vi "DAQ.44xx.Get Ref Clk.vi"(8 "error in (no error)":errorcluster, 11 "Refnum in":refnum<k21>) -> (0 "error out":errorcluster, 2 "RefClk.Src":tag, 3 "Refnum out":refnum<k21>)   [LabVIEW 2019, in "Instrument.Lockin.lvlib" / "Instrument.DAQ.lvclass"]
uses:
  Instrument.DAQ.lvclass
  <resource>/objmgr/daqmx.rc
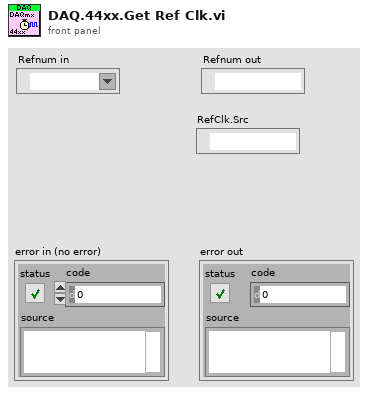
[diagram p1: front panel]
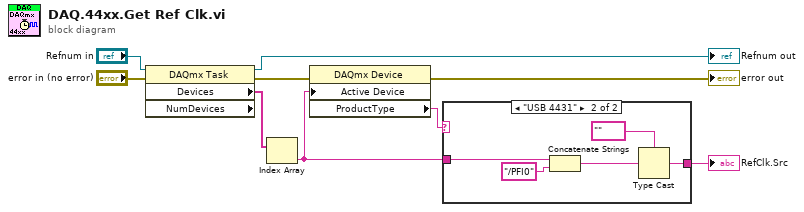
[diagram p0: block diagram]
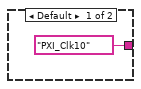
[diagram p2: hidden frame]
diagram:
  n1 = property class="DAQmx Task" props=["Devices", "NumDevices"](reference="Refnum in", error in="error in (no error)") -> (reference out=→"Refnum out":refnum<k21>, error out=w4:errorcluster, "Devices"=w8:tag[])  [unwired: 1 out]
  n2 = Index Array(array=w8) -> (element=w5:tag)  [unwired: 1 in]
  n3 = property class="DAQmx Device"(error in=w4, "Active Device"=w5) -> (error out=→"error out":errorcluster, "ProductType"=w3:string)  [unwired: 1 in, 1 out]
  n4 = case shown="\"USB 4431\"" w3 {
    tunnel: [tag "PXI_Clk10" ("RefClk.Src") w12] -> w9
    tunnel: w5 -> [_ w11]
    frame Default {
    }
    frame "USB 4431" {
      n5 = Concatenate Strings(w11, "/PFI0" ("string")) -> (w13:string)
      n6 = Type Cast(type=tag "" ("RefClk.Src"), x=w13) -> (*(type *) &x=w12:tag)
    }
  }
  "RefClk.Src" <- w9
